vi "BuildFarm INI Tool.vi"(7 "WorkerShow":bool=TRUE, 8 "error in (no error)":errorcluster, 9 "CommPort":u32=4545, 10 "WorkerFolder":path=path "/Volumes/Data/Users/benji667/Git/BuildFarm/src/BuildWorker", 11 "WorkerInterface":string="BuildWorker Basics.lvclass") -> (0 "error out":errorcluster, 3 "file path":path)   [LabVIEW 2017]
uses:
  <vilib>/Utility/config.llb/Write Key (String).vi
  <vilib>/Utility/config.llb/Write Key (Path).vi
  <vilib>/Utility/config.llb/Write Key (Boolean).vi
  <vilib>/Utility/config.llb/Write Key (U32).vi
  <vilib>/Utility/config.llb/NI_LVConfig.lvlib
panel:
  in  "ServerFolder":path=path "/Volumes/Data/Users/benji667/Git/BuildFarm/src/BuildServer"
  in  "ServerLauncher":string="BuildServer Launcher.vi"
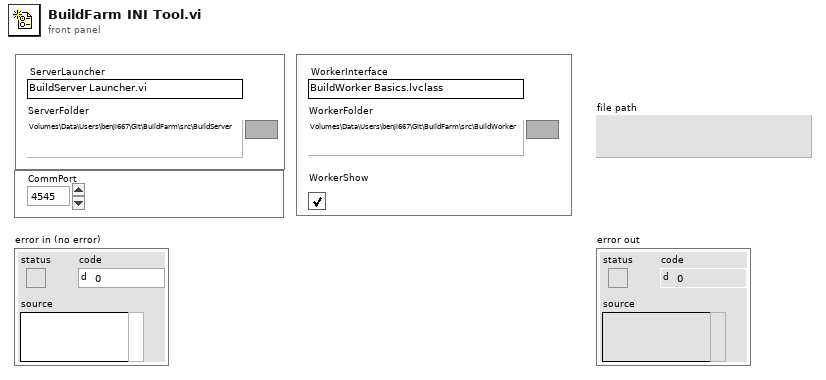
[diagram p1: front panel]
types:
  T1 = typedef "NI_LVConfig.lvlib/Config Data RefNum.ctl" = refnum<k1>
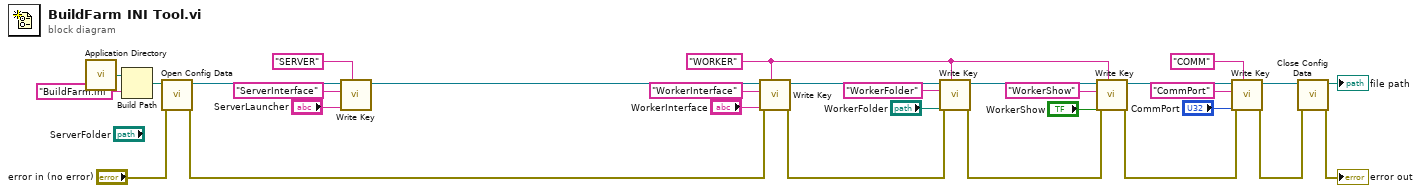
[diagram p0: block diagram]
diagram:
  w12 = "WORKER" ("section")
  n1 = call <vilib>:"Application Directory.vi"() -> ("Application Directory"=w30:path)
  n2 = Build Path(base path=w30, name or relative path="BuildFarm.ini") -> (appended path=w11:path)
  n3 = call <vilib>:"Open Config Data.vi"("error in (no error)"="error in (no error)", "configuration file path"=w11) -> ("error out"=w28:errorcluster, "refnum"=w2:T1)  [unwired: 7 in, 1 out]
  n4 = call-poly <vilib>:"Write Key.vi"("section"="SERVER", "value"="ServerLauncher", "key"="ServerInterface", "refnum"=w2) -> ("refnum out"=w1:T1)  [unwired: 5 in, 2 out]
  n5 = call-poly <vilib>:"Write Key.vi"("section"=w12, "error in (no error)"=w28, "value"="WorkerInterface", "key"="WorkerInterface", "refnum"=w1) -> ("error out"=w14:errorcluster, "refnum out"=w17:T1)  [unwired: 4 in, 1 out]
  n6 = call-poly <vilib>:"Write Key.vi"("section"=w12, "error in (no error)"=w14, "value"="WorkerFolder", "key"="WorkerFolder", "refnum"=w17) -> ("error out"=w13:errorcluster, "refnum out"=w16:T1)  [unwired: 4 in, 1 out]
  n7 = call-poly <vilib>:"Write Key.vi"("section"=w12, "error in (no error)"=w13, "value"="WorkerShow", "key"="WorkerShow", "refnum"=w16) -> ("error out"=w22:errorcluster, "refnum out"=w23:T1)  [unwired: 4 in, 1 out]
  n8 = call-poly <vilib>:"Write Key.vi"("section"="COMM", "error in (no error)"=w22, "value"="CommPort", "key"="CommPort", "refnum"=w23) -> ("error out"=w20:errorcluster, "refnum out"=w21:T1)  [unwired: 4 in, 1 out]
  n9 = call <vilib>:"Close Config Data.vi"("error in (no error)"=w20, "refnum"=w21) -> ("error out"=→"error out":errorcluster, "file path"=→"file path":path)  [unwired: 8 in]
